vi "Apply Properties from Configuration File.vi"(4 "String Properties":string[](array[string]), 6 "Boolean Properties":string[](array[string]), 7 "Numeric Properties":string[](array[string]), 8 "error in":errorcluster, 9 "Section":string, 10 "Configuration File Path":path, 11 "Item Reference In":T1 format="%.0x") -> (0 "error out":errorcluster, 3 "Item Device Reference Out":T1 format="%.0x")   [LabVIEW 2027, in "Embedded Data Logger System Explorer.lvlib"]
uses:
  Embedded Data Logger System Explorer.lvlib
  <vilib>/NI VeriStand/Custom Device API/Custom Device Item Ref.ctl
  <vilib>/Utility/config.llb/Read Key (String).vi
  <vilib>/NI VeriStand/Custom Device API/Set Item Property (String).vi
  <vilib>/Utility/config.llb/Read Key (Double).vi
  <vilib>/NI VeriStand/Custom Device API/Set Item Property (Double).vi
  <vilib>/Utility/config.llb/Read Key (Boolean).vi
  <vilib>/NI VeriStand/Custom Device API/Set Item Property (Boolean).vi
  <vilib>/Utility/config.llb/NI_LVConfig.lvlib
  <vilib>/NI VeriStand/Custom Device API/Custom Device API.lvlib
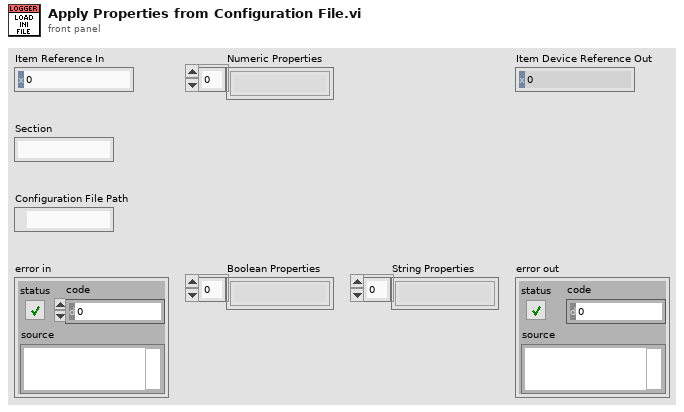
[diagram p1: front panel]
types:
  T1 = typedef "Custom Device API.lvlib/Custom Device Item Ref.ctl" = u64
  T2 = typedef "NI_LVConfig.lvlib/Config Data RefNum.ctl" = refnum<k1>
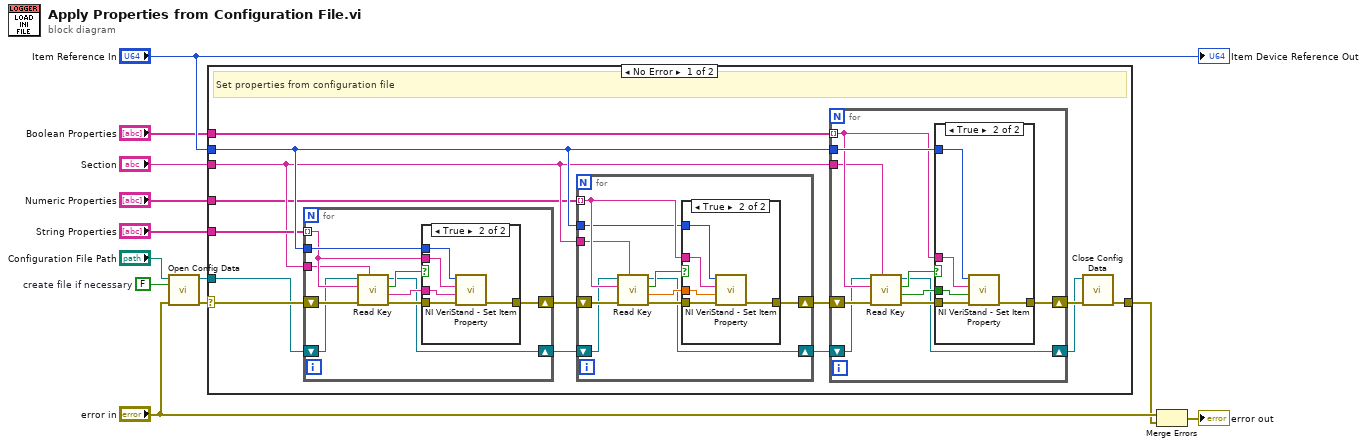
[diagram p0: block diagram]
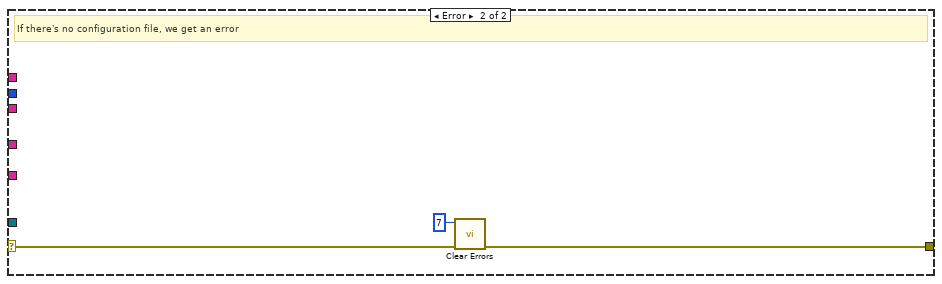
[diagram p5: hidden frame]
diagram:
  w7 = FALSE  # create file if necessary
  n1 = call <vilib>:"Open Config Data.vi"("error in (no error)"="error in", "create file if necessary (T)"=w7, "configuration file path"="Configuration File Path") -> ("error out"=w5:errorcluster, "refnum"=w6:T2)  [unwired: 6 in, 1 out]
  n2 = case shown="No Error" w5 {
    selector: w5 -> [w17 w77]
    tunnel: "Item Reference In" -> [w24 _]
    tunnel: "String Properties" -> [w21 _]
    tunnel: "Section" -> [w20 _]
    tunnel: "Numeric Properties" -> [w19 _]
    tunnel: "Boolean Properties" -> [w18 _]
    tunnel: w6 -> [w16 _]
    tunnel: [w13 w76] -> w1
    frame No Error {
      # "Set properties from configuration file"
      n3 = for {
        shift-right: [w35] -> w26
        shift-left: w17 -> [w36]
        tunnel: w21 -> [w30] mode=indexing
        tunnel: w24 -> [w31]
        shift-right: [w28] -> w23
        shift-left: w16 -> [w29]
        tunnel: w20 -> [w27]
        n4 = call-poly <vilib>:"Read Key.vi"("section"=w27, "error in (no error)"=w36, "key"=w30, "refnum"=w29) -> ("error out"=w34:errorcluster, "value"=w32:string, "found?"=w33:bool, "refnum out"=w28:T2)  [unwired: 4 in]
        n5 = case shown="True" w33 {
          tunnel: w34 -> [w37 w42]
          tunnel: [w37 w41] -> w35
          tunnel: w32 -> [_ w40]
          tunnel: w31 -> [_ w39]
          tunnel: w30 -> [_ w38]
          frame False {
          }
          frame True {
            n6 = call-poly <vilib>:"NI VeriStand - Set Item Property.vi"("error in (no error)"=w42, "Value"=w40, "Property Name"=w38, "Item Ref in"=w39) -> ("error out"=w41:errorcluster)  [unwired: 5 in, 2 out]
          }
        }
      }
      n7 = for {
        shift-right: [w67] -> w25
        shift-left: w26 -> [w68]
        tunnel: w19 -> [w63] mode=indexing
        tunnel: w24 -> [w62]
        shift-right: [w60] -> w22
        shift-left: w23 -> [w61]
        tunnel: w20 -> [w59]
        n8 = call-poly <vilib>:"Read Key.vi"("section"=w59, "error in (no error)"=w68, "key"=w63, "refnum"=w61) -> ("error out"=w66:errorcluster, "value"=w64:dbl, "found?"=w65:bool, "refnum out"=w60:T2)  [unwired: 4 in]
        n9 = case shown="True" w65 {
          tunnel: w66 -> [w69 w74]
          tunnel: [w69 w73] -> w67
          tunnel: w64 -> [_ w72]
          tunnel: w63 -> [_ w71]
          tunnel: w62 -> [_ w70]
          frame False {
          }
          frame True {
            n10 = call-poly <vilib>:"NI VeriStand - Set Item Property.vi"("error in (no error)"=w74, "Value"=w72, "Property Name"=w71, "Item Ref in"=w70) -> ("error out"=w73:errorcluster)  [unwired: 5 in, 2 out]
          }
        }
      }
      n11 = for {
        shift-right: [w51] -> w15
        shift-left: w25 -> [w52]
        tunnel: w18 -> [w46] mode=indexing
        tunnel: w24 -> [w47]
        shift-right: [w44] -> w14
        shift-left: w22 -> [w45]
        tunnel: w20 -> [w43]
        n12 = call-poly <vilib>:"Read Key.vi"("section"=w43, "error in (no error)"=w52, "key"=w46, "refnum"=w45) -> ("error out"=w50:errorcluster, "value"=w48:bool, "found?"=w49:bool, "refnum out"=w44:T2)  [unwired: 4 in]
        n13 = case shown="True" w49 {
          tunnel: w50 -> [w53 w58]
          tunnel: [w53 w57] -> w51
          tunnel: w48 -> [_ w56]
          tunnel: w47 -> [_ w54]
          tunnel: w46 -> [_ w55]
          frame False {
          }
          frame True {
            n14 = call-poly <vilib>:"NI VeriStand - Set Item Property.vi"("error in (no error)"=w58, "Value"=w56, "Property Name"=w55, "Item Ref in"=w54) -> ("error out"=w57:errorcluster)  [unwired: 5 in, 2 out]
          }
        }
      }
      n15 = call <vilib>:"Close Config Data.vi"("error in (no error)"=w15, "refnum"=w14) -> ("error out"=w13:errorcluster)  [unwired: 8 in, 1 out]
    }
    frame Error {
      # "If there's no configuration file, we get an error"
      n16 = call <vilib>:"Clear Errors.vi"("error in (no error)"=w77, "specific error code to clear (0: all)"=7) -> ("error out"=w76:errorcluster)  [unwired: 4 in, 1 out]
    }
  }
  n17 = Merge Errors("error in", w1) -> (→"error out":errorcluster)
  "Item Device Reference Out" <- "Item Reference In"
